vi "GetBlockStopPos.vi"(9 "YB":dbl, 11 "XB":dbl) -> (1 "Array B":dbl[](array[numeric]), 3 "Array":dbl[](array[numeric]))   [LabVIEW 2018]
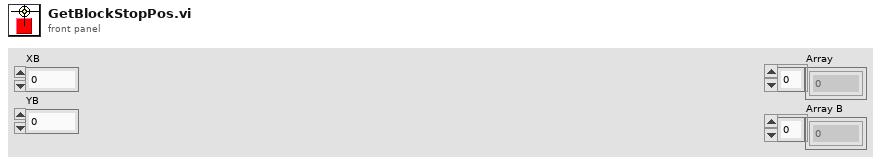
[diagram p1: front panel]
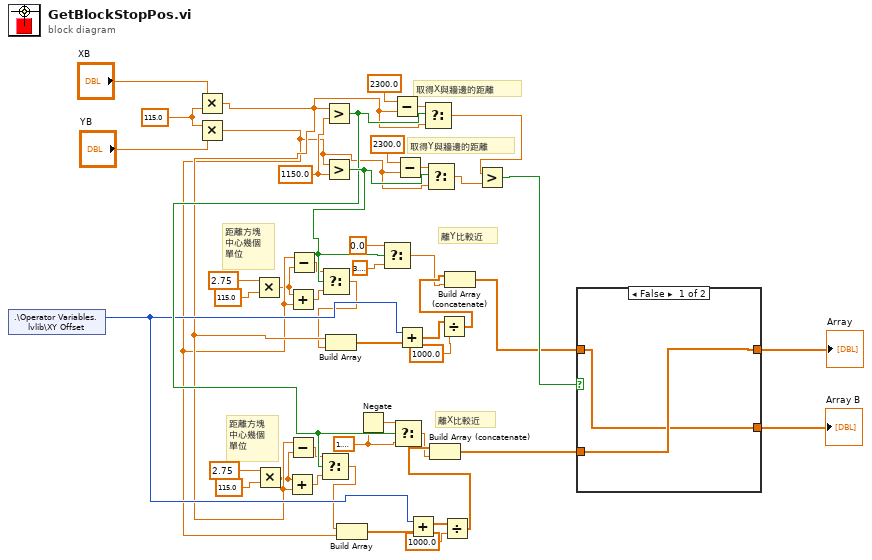
[diagram p0: block diagram]
diagram:
  w7 = 1.5707963267948966
  w39 = 115.0
  w40 = 1150.0 ("y")
  # "距離方塊\n中心幾個\n單位"
  # "離X比較近"
  # "距離方塊\n中心幾個\n單位"
  # "離Y比較近"
  # "取得Y與牆邊的距離"
  # "取得X與牆邊的距離"
  n1 = shared-variable ".\\Operator Variables.lvlib\\XY Offset"() -> (w34:i16)  [unwired: 1 in, 1 out]
  n2 = Multiply(x="XB", y=w39) -> (x*y=w33:dbl)
  n3 = Multiply(x=w39, y="YB") -> (x*y=w32:dbl)
  n4 = Multiply(x=2.75 ("y"), y=115.0) -> (x*y=w20:dbl)
  n5 = Multiply(x=2.75 ("y"), y=115.0) -> (x*y=w9:dbl)
  n6 = Add(x=w9, y=w33) -> (x+y=w17:dbl)
  n7 = Add(x=w20, y=w32) -> (x+y=w30:dbl)
  n8 = Subtract(x=w33, y=w9) -> (x-y=w18:dbl)
  n9 = Subtract(x=w32, y=w20) -> (x-y=w31:dbl)
  n10 = Greater?(x=w33, y=w40) -> (0:w35:bool)
  n11 = Select(t=w18, s=w35, f=w17) -> (s? t:f=w13:dbl)
  n12 = Greater?(x=w32, y=w40) -> (0:w46:bool)
  n13 = Select(t=w31, s=w46, f=w30) -> (s? t:f=w26:dbl)
  n14 = Build Array(w33, w26) -> (w23:dbl[])
  n15 = Build Array(w13, w32) -> (w6:dbl[])
  n16 = Negate(x=w7) -> (-x=w8:dbl)
  n17 = Select(t=0.0, s=w46, f=3.141592653589793) -> (s? t:f=w24:dbl)
  n18 = Subtract(x=2300.0, y=w33) -> (x-y=w43:dbl)
  n19 = Select(t=w8, s=w35, f=w7) -> (s? t:f=w12:dbl)
  n20 = Subtract(x=2300.0, y=w32) -> (x-y=w44:dbl)
  n21 = Add(x=w34, y=w23) -> (x+y=w29:dbl[])
  n22 = Add(x=w34, y=w6) -> (x+y=w16:dbl[])
  n23 = Select(t=w43, s=w35, f=w33) -> (s? t:f=w38:dbl)
  n24 = Select(t=w44, s=w46, f=w32) -> (s? t:f=w45:dbl)
  n25 = Divide(x=w29, y=1000.0) -> (x/y=w25:dbl[])
  n26 = Divide(x=w16, y=1000.0) -> (x/y=w14:dbl[])
  n27 = Build Array (concatenate)(w14, w12) -> (w2:dbl[])
  n28 = Build Array (concatenate)(w25, w24) -> (w3:dbl[])
  n29 = Greater?(x=w38, y=w45) -> (0:w5:bool)
  n30 = case shown="False" w5 {
    tunnel: [w48 w50] -> w4
    tunnel: w3 -> [w47 w50]
    tunnel: w2 -> [w48 w49]
    tunnel: [w47 w49] -> w1
    frame False {
    }
    frame True {
    }
  }
  "Array" <- w4
  "Array B" <- w1
